vi "Update.vi"(8 "error in (no error)":errorcluster, 11 "LoggingControl in":refnum<class "LoggingControl.lvclass">) -> (0 "error out":errorcluster, 3 "LoggingControl out":refnum<class "LoggingControl.lvclass">)   [LabVIEW 2020, in "VolatusGUIElements.lvlib" / "LoggingControl.lvclass"]
uses:
  LoggingControl.lvclass
  C:/dev/lv20CE/relink/lv-volatus/VolatusGUI/GUI Element/GUI Element.lvclass
  LoggingControl.lvclass/LoggingControl.ctl
  <vilib>/Utility/miscctls.llb/LVMapReplaceAction.ctl
  lv-vecto/Vecto/Channel DBL/Channel DBL.lvclass/Channel DBL.ctl
  VolatusGUI/GUI Element/GUI Element.lvclass/GUI Element.ctl
  lv-vecto/Vecto/Group DBL/Value by Index.vi
  lv-vecto/Vecto/Channel DBL/Channel DBL.lvclass
  Volatus/VolatusAPI/VolatusAPI.lvclass
  <vilib>/httpClient/LabVIEWHTTPClient.lvlib
  VolatusGUI/GUI Element/GUI Element.lvclass
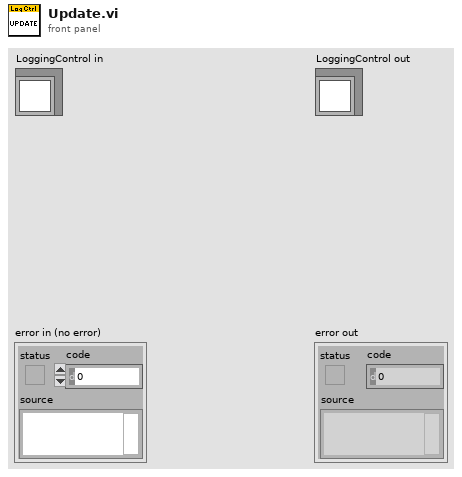
[diagram p1: front panel]
types:
  T1 = typedef "LVMapReplaceAction.ctl" = enum32{"Modify Entry only if found", "Add or Modify Entry", "Delete Entry"}
  T2 = cluster{string, string, "All Logging":bool, cluster{"String":string, u32, "State":string}[]}
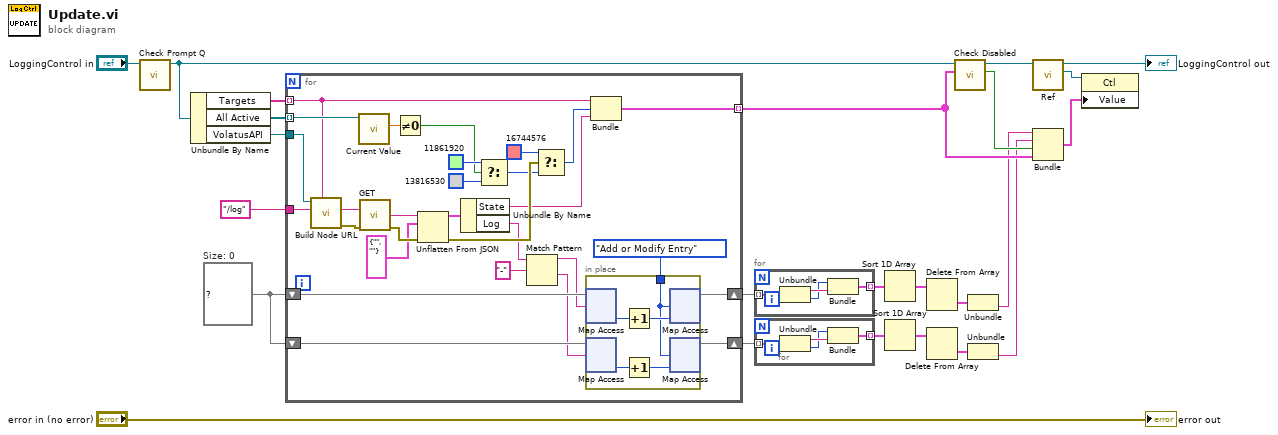
[diagram p0: block diagram]
diagram:
  w11 = map{string, i32} {}  # Size: 0
  n1 = call "Check Prompt Q.vi"("LoggingControl in"="LoggingControl in") -> ("LoggingControl out"=w22:refnum<class "LoggingControl.lvclass">)  [unwired: 9 in, 1 out]
  n2 = Unbundle By Name(w22) -> ("Targets"=w23:string[], "All Active"=w18:refnum<class "Channel DBL.lvclass">[], "VolatusAPI"=w17:refnum<class "VolatusAPI.lvclass">)
  n3 = for {
    tunnel: w23 -> [w41] mode=indexing
    tunnel: [w46] -> w21 mode=indexing
    tunnel: w18 -> [w44] mode=indexing
    tunnel: w17 -> [w42]
    tunnel: "/log" -> [w40]
    shift-right: [w33] -> w10
    shift-left: w11 -> [w30]
    shift-right: [w32] -> w2
    shift-left: w11 -> [w31]
    n4 = call "Build Node URL.vi"("Node Name"=w41, "Path"=w40, "VolatusAPI in"=w42) -> ("error out"=w37:errorcluster, "Request URL"=w39:string)  [unwired: 6 in, 1 out]
    n5 = call "Current Value.vi"("Channel in"=w44) -> ("Scaled"=w45:dbl)  [unwired: 6 in, 4 out]
    n6 = call <vilib>:"GET.vi"("url"=w39, "error in (no error)"=w37) -> ("body"=w38:string, "error out"=w52:errorcluster)  [unwired: 10 in, 2 out]
    n7 = Not Equal To 0?(x=w45) -> (x != 0?=w43:bool)
    n8 = Unflatten From JSON(JSON string=w38, type and defaults=cluster{"State":string, "Log":string} {"State"="", "Log"=""} ("output cluster"), error in (no error)=w52) -> (value=w35:cluster{"State":string, "Log":string}, error out=w53:errorcluster)  [unwired: 4 in]
    n9 = Unbundle By Name(w35) -> ("State"=w34:string, "Log"=w29:string)
    n10 = Select(t=u32 11861920, s=w43, f=u32 13816530) -> (s? t:f=w49:u32)
    n11 = Match Pattern(string=w29, regular expression="-") -> (before substring=w27:string, after substring=w26:string)  [unwired: 1 in, 2 out]
    n12 = Select(t=u32 16744576, s=w53, f=w49) -> (s? t:f=w47:u32)
    n13 = in-place {
      in-place-border: LVMapReplaceAction."Add or Modify Entry" ("action") -> [w54]
      n14 = in-place-map #1(w30, w27) -> (w58:i32)  [unwired: 1 in, 1 out]
      n15 = in-place-map #2(w31, w26) -> (w57:i32)  [unwired: 1 in, 1 out]
      n16 = Increment(x=w58) -> (x+1=w55:i32)
      n17 = Increment(x=w57) -> (x+1=w56:i32)
      n18 = in-place-map #1(w55, w54) -> (w33:map{string, i32})  [unwired: 2 out]
      n19 = in-place-map #2(w56, w54) -> (w32:map{string, i32})  [unwired: 2 out]
    }
    n20 = Bundle("String"=w41, w47, "State"=w34) -> (w46:cluster{"String":string, u32, "State":string})  [unwired: 1 in]
  }
  n21 = for {
    tunnel: w10 -> [w62] mode=indexing
    tunnel: [w59] -> w9 mode=indexing
    n22 = Unbundle(w62) -> (w61:string, w60:i32)
    n23 = Bundle(w60, w61) -> (w59:cluster{i32, string})  [unwired: 1 in]
  }
  n24 = for {
    tunnel: w2 -> [w66] mode=indexing
    tunnel: [w63] -> w3 mode=indexing
    n25 = Unbundle(w66) -> (w65:string, w64:i32)
    n26 = Bundle(w64, w65) -> (w63:cluster{i32, string})  [unwired: 1 in]
  }
  n27 = Sort 1D Array(array=w9) -> (sorted array=w8:cluster{i32, string}[])
  n28 = Sort 1D Array(array=w3) -> (sorted array=w4:cluster{i32, string}[])
  n29 = Delete From Array(array=w8) -> (deleted portion=w7:cluster{i32, string})  [unwired: 2 in, 1 out]
  n30 = Delete From Array(array=w4) -> (deleted portion=w5:cluster{i32, string})  [unwired: 2 in, 1 out]
  n31 = call "Check Disabled.vi"("Array"=w21, "LoggingControl in"=w22) -> ("All Logging"=w15:bool, "LoggingControl out"=w19:refnum<class "LoggingControl.lvclass">)  [unwired: 7 in, 1 out]
  n32 = Unbundle(w7) -> (w6:string)  [unwired: 1 out]
  n33 = Unbundle(w5) -> (w1:string)  [unwired: 1 out]
  n34 = call "Ref.vi"("GUI Element in"=w19) -> ("Ref"=w13:refnum<vi>, "GUI Element out"=→"LoggingControl out":refnum<class "LoggingControl.lvclass">)  [unwired: 9 in]
  n35 = Bundle(w6, w1, "All Logging"=w15, w21) -> (w12:T2)  [unwired: 1 in]
  n36 = property class="Ctl"(reference=w13, "Value"=w12) -> ()  [unwired: 1 in, 2 out]
  "error out" <- "error in (no error)"
